vi "Default Path.vi"(8 "error in (no error)":errorcluster, 11 "OpenSSH Client in":refnum<class "OpenSSH Client.lvclass">) -> (0 "error out":errorcluster, 2 "path":path, 3 "OpenSSH Client out":refnum<class "OpenSSH Client.lvclass">)   [LabVIEW 2020, in "NI_SSH.lvlib" / "OpenSSH Client.lvclass"]
uses:
  <vilib>/net/SSH/Client/OpenSSH/OpenSSH Client.lvclass
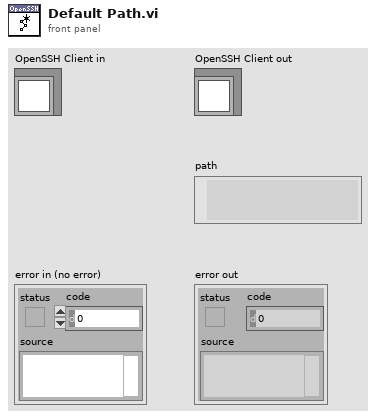
[diagram p1: front panel]
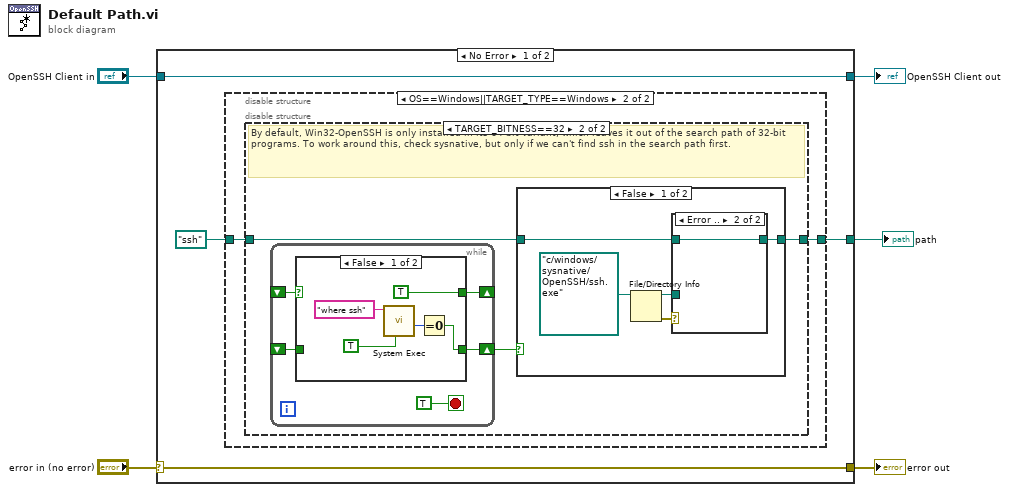
[diagram p0: block diagram]
diagram:
  n1 = case shown="No Error" "error in (no error)" {
    selector: "error in (no error)" -> [w8 w38]
    tunnel: [w8 w38] -> w4
    tunnel: [w9 w37] -> w2
    tunnel: "OpenSSH Client in" -> [w9 w37]
    tunnel: [w6 _] -> w1
    frame No Error {
      n2 = disable-structure "Conditional Disable Structure" shown="OS==Windows||TARGET_TYPE==Windows" {
        disable-tunnel: [w10 w11] -> w6
        disable-tunnel: path "ssh" ("path") -> [w10 w12]
        frame condition #0 {
        }
        frame condition #1 (active) {
          n3 = disable-structure "Conditional Disable Structure" shown="TARGET_BITNESS==32" {
            disable-tunnel: w12 -> [w13 w14]
            disable-tunnel: [w13 w16] -> w11
            frame condition #0 {
            }
            frame condition #1 (active) {
              # "By default, Win32-OpenSSH is only installed in its 64-bit variant, which leaves it out of the search path of 32-bit programs. To work around this, check sysnative, but only if we can't find ssh in the search path first."
              n4 = while {
                shift-right: [w29] -> _
                shift-left: _ -> [w28]
                shift-right: [w27] -> w15
                shift-left: _ -> [w26]
                stop <- TRUE stop-if-true
                n5 = case shown="False" w28 {
                  selector: w28 -> [_ w35]
                  tunnel: [TRUE w35] -> w29
                  tunnel: [w31 w36] -> w27
                  tunnel: w26 -> [_ w36]
                  frame False {
                    n6 = call <vilib>:"System Exec.vi"("run minimized? (F)"=TRUE, "command line"="where ssh" ("format string")) -> ("return code"=w32:i32)  [unwired: 6 in, 3 out]
                    n7 = Equal To 0?(x=w32) -> (x = 0?=w31:bool)
                  }
                  frame True {
                  }
                }
              }
              n8 = case shown="False" w15 {
                tunnel: [w18 w24] -> w16
                tunnel: w14 -> [w17 w24]
                frame False {
                  n9 = File/Directory Info(path=path "c:/windows/sysnative/OpenSSH/ssh.exe") -> (path out=w19:path, error out=w20:errorcluster)  [unwired: 1 in, 5 out]
                  n10 = case shown="Error .." w20 {
                    tunnel: w19 -> [w22 _]
                    tunnel: [w22 w23] -> w18
                    tunnel: w17 -> [_ w23]
                    frame No Error {
                    }
                    frame Error {
                      # "give up"
                    }
                  }
                }
                frame True {
                }
              }
            }
          }
        }
      }
    }
    frame Error {
    }
  }
  "error out" <- w4
  "OpenSSH Client out" <- w2
  "path" <- w1
